vi "Extract Newest Data.vi"(6 "Triggered?":bool, 8 "Error in":errorcluster, 9 "Filtered Signal":dbl[](array[numeric]), 10 "Raw Signal":dbl[](array[numeric]), 11 "State Variables in":T1={"Stop Notifier"=refnum, "UI References"=[], "DAQmx"={"ECG Input"={"Channel"="", "Task"="", "Max Value"=0.0, "Min Value"=0.0, "Sampling Rate"=0.0, "Batch Size"=0}, "Trigger Output"={"Channel"="", "Task"="", "Pulse Frequency"=0.0, "Delay"=0, "Triggers per Shot"=0}}, "Data Queue"=refnum, "Filter"={"Batch Size"=1000, "Update Cycle"=0, "Filter Buffer"=[]}, "Last Detect Result"=FALSE}) -> (0 "Error out":errorcluster, 2 "Chart out":dbl[][](array[numeric]), 3 "State Variables out":T1={"Stop Notifier"=refnum, "UI References"=[], "DAQmx"={"ECG Input"={"Channel"="", "Task"="", "Max Value"=0.0, "Min Value"=0.0, "Sampling Rate"=0.0, "Batch Size"=0}, "Trigger Output"={"Channel"="", "Task"="", "Pulse Frequency"=0.0, "Delay"=0, "Triggers per Shot"=0}}, "Data Queue"=refnum, "Filter"={"Batch Size"=1000, "Update Cycle"=0, "Filter Buffer"=[]}, "Last Detect Result"=FALSE})   [LabVIEW 2014, in "Filter.lvlib"]
uses:
  Filter.lvlib
  Controls/State Variables.ctl
  Controls/DAQmx Variables.ctl
  Controls/Filter Variables.ctl
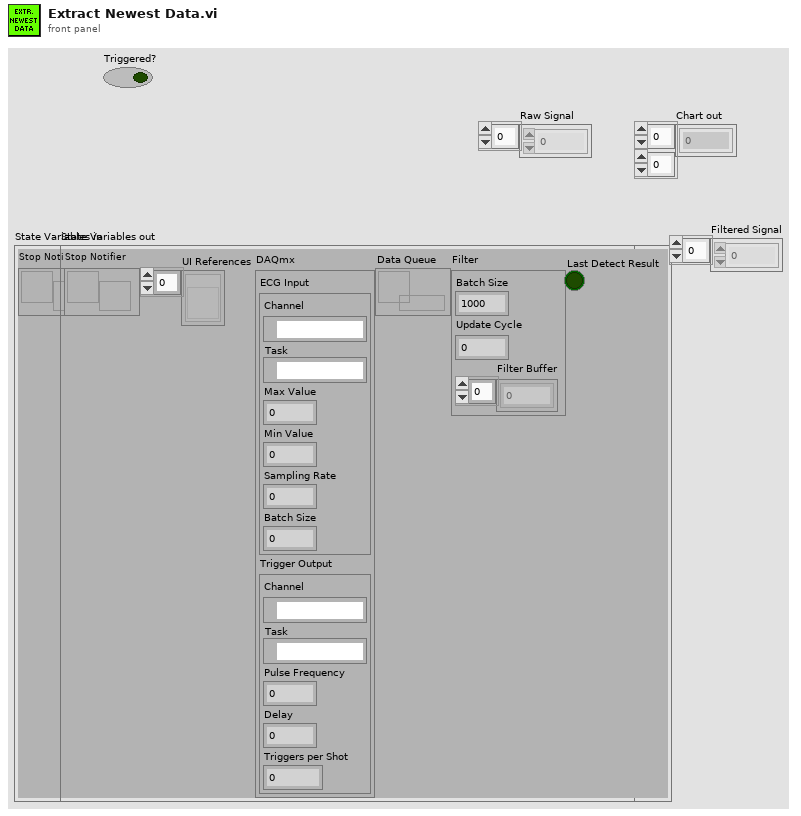
[diagram p1: front panel]
types:
  T1 = typedef "State Variables.ctl" = cluster{"Stop Notifier":refnum<notifier>, "UI References":refnum<vi>[], "DAQmx":T2, "Data Queue":refnum<queue>, "Filter":T3, "Last Detect Result":bool}
  T2 = typedef "DAQmx Variables.ctl" = cluster{"ECG Input":cluster{"Channel":tag, "Task":refnum<k21>, "Max Value":dbl, "Min Value":dbl, "Sampling Rate":dbl, "Batch Size":i32}, "Trigger Output":cluster{"Channel":tag, "Task":refnum<k21>, "Pulse Frequency":dbl, "Delay":u16, "Triggers per Shot":i32}}
  T3 = typedef "Filter Variables.ctl" = cluster{"Batch Size":i32, "Update Cycle":i32, "Filter Buffer":dbl[]}
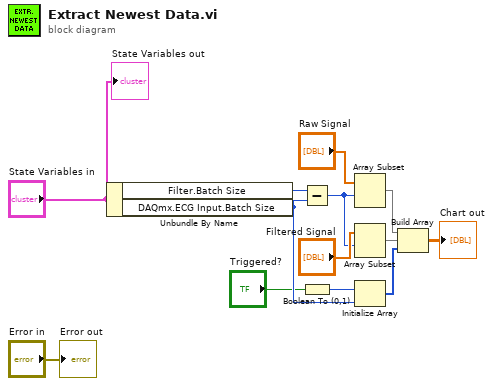
[diagram p0: block diagram]
diagram:
  n1 = Unbundle By Name("State Variables in") -> ("Filter.Batch Size"=w12:i32, "DAQmx.ECG Input.Batch Size"=w2:i32)
  n2 = Subtract(x=w12, y=w2) -> (x-y=w6:i32)
  n3 = Boolean To (0,1)(Boolean="Triggered?") -> (0, 1=w3:i16)
  n4 = Array Subset(array="Raw Signal", index=w6) -> (w8:dbl[])  [unwired: 1 in]
  n5 = Array Subset(array="Filtered Signal", index=w6) -> (w7:dbl[])  [unwired: 1 in]
  n6 = Initialize Array(w3, w2) -> (w4:i16[])
  n7 = Build Array(w8, w7, w4) -> (→"Chart out":dbl[][])
  "Error out" <- "Error in"
  "State Variables out" <- "State Variables in"
